vi "Save for Previous Version (vi).vi"(6 "Destination Folder":path, 7 "Folder to Convert":path, 8 "error in (no error)":errorcluster, 9 "Show Front Panel?":bool, 10 "Previous Version":string(combo), 11 "vi path":path) -> (0 "error out":errorcluster, 2 "Warnings":string)   [LabVIEW 2023]
panel:
  out "vi path 2":path
  out "appended path":path
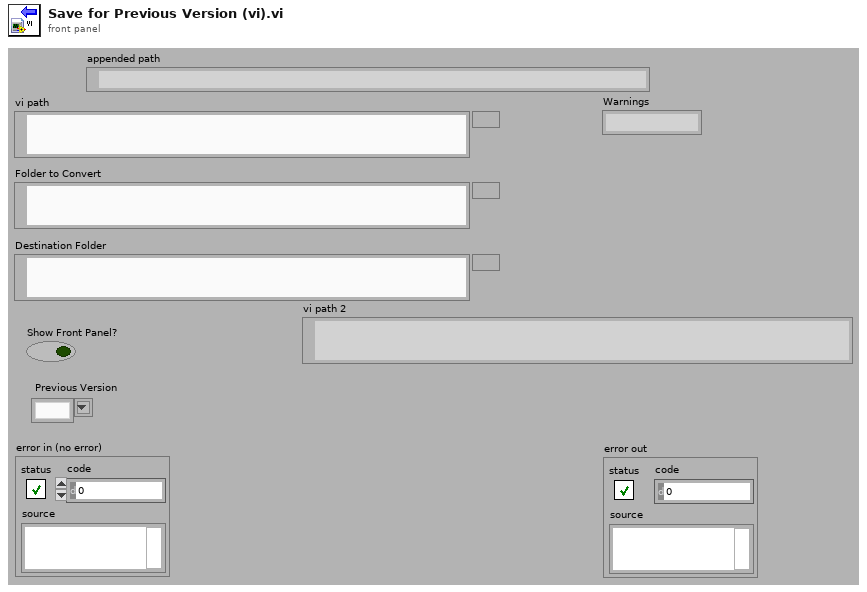
[diagram p1: front panel]
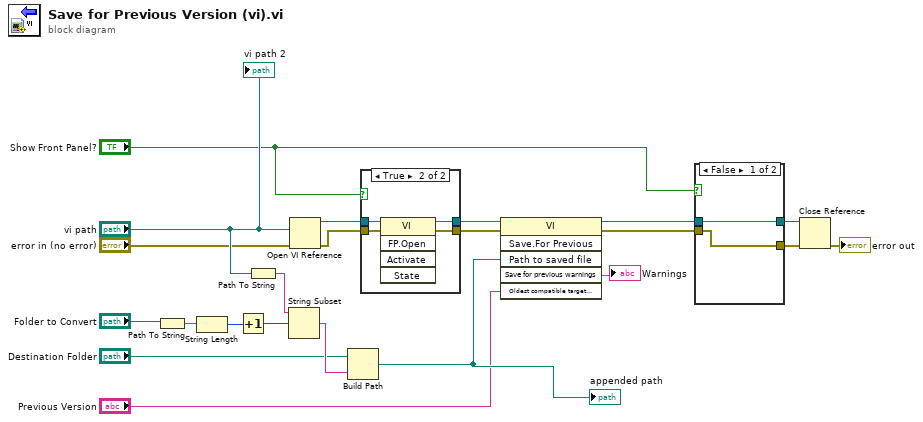
[diagram p0: block diagram]
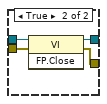
[diagram p2: hidden frame]
diagram:
  n1 = Path To String(path="Folder to Convert") -> (string=w5:string)
  n2 = String Length(string=w5) -> (length=w4:i32)
  n3 = Increment(x=w4) -> (x+1=w2:i32)
  n4 = Path To String(path="vi path") -> (string=w16:string)
  n5 = String Subset(string=w16, offset (0)=w2) -> (substring=w17:string)  [unwired: 1 in]
  n6 = Open VI Reference(vi path="vi path", error in (no error)="error in (no error)") -> (vi reference=w22:refnum<vi>, error out=w21:errorcluster)  [unwired: 4 in]
  n7 = Build Path(base path="Destination Folder", name or relative path=w17) -> (appended path=w15:path)
  "appended path" <- w15
  n8 = case shown="True" "Show Front Panel?" {
    tunnel: w22 -> [w24 w28]
    tunnel: w21 -> [w23 w27]
    tunnel: [w24 w26] -> w20
    tunnel: [w23 w25] -> w19
    frame False {
    }
    frame True {
      n9 = invoke class="VI" method="FP.Open"(reference=w28, error in=w27) -> (reference out=w26:refnum<vi>, error out=w25:errorcluster)  [unwired: 3 in, 3 out]
    }
  }
  n10 = invoke class="VI" method="Save.For Previous"(reference=w20, error in=w19, "Path to saved file"=w15, "Oldest compatible target version"="Previous Version") -> (reference out=w14:refnum<vi>, error out=w13:errorcluster, "Save for previous warnings"=→"Warnings":string)  [unwired: 2 in, 3 out]
  n11 = case shown="False" "Show Front Panel?" {
    tunnel: w14 -> [w30 w34]
    tunnel: w13 -> [w29 w33]
    tunnel: [w30 w32] -> w11
    tunnel: [w29 w31] -> w10
    frame False {
    }
    frame True {
      n12 = invoke class="VI" method="FP.Close"(reference=w34, error in=w33) -> (reference out=w32:refnum<vi>, error out=w31:errorcluster)  [unwired: 1 in, 1 out]
    }
  }
  n13 = Close Reference(reference=w11, error in (no error)=w10) -> (error out=→"error out":errorcluster)
  "vi path 2" <- "vi path"
